vi "SetMeasBand.vi"(6 "Legacy (f)?":bool, 8 "error in (no error)":errorcluster, 10 "Band Index":u32) -> (0 "error out":errorcluster)   [LabVIEW 2011]
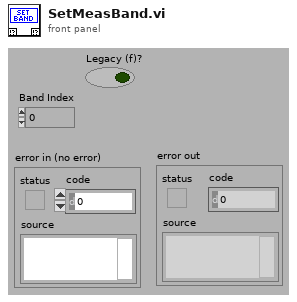
[diagram p1: front panel]
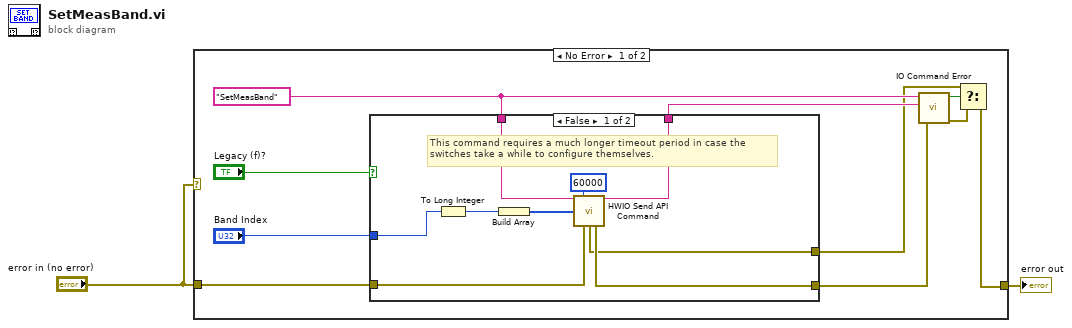
[diagram p0: block diagram]
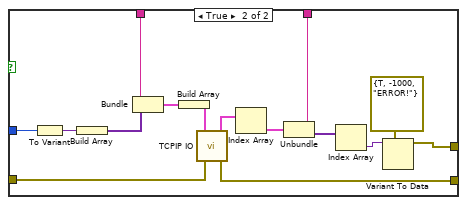
[diagram p2: hidden frame]
diagram:
  n1 = case shown="No Error" "error in (no error)" {
    tunnel: "error in (no error)" -> [w11 w37]
    tunnel: [w4 w37] -> w2
    frame No Error {
      w9 = "SetMeasBand"
      n2 = case shown="False" "Legacy (f)?" {
        tunnel: "Band Index" -> [w21 w36]
        tunnel: w11 -> [w20 w33]
        tunnel: [w19 w31] -> w10
        tunnel: w9 -> [w17 w30]
        tunnel: [w18 w26] -> w8
        tunnel: [w14 w23] -> w5
        frame False {
          # "This command requires a much longer timeout period in case the\nswitches take a while to configure themselves."
          n3 = To Long Integer(number=w21) -> (32bit integer=w15:i32)
          n4 = Build Array(w15) -> (w16:i32[])
          n5 = call "HWIO Send API Command.vi"("Action"=w17, "Timeout ms (5000)"=60000 ("Timeout ms (10000)"), "Integer"=w16, "error in (no error)"=w20) -> ("Action out"=w18:string, "HWError"=w14:errorcluster, "error out"=w19:errorcluster)  [unwired: 4 in, 5 out]
        }
        frame True {
          n6 = To Variant(anything=w36) -> (Variant=w35:variant)
          n7 = Build Array(w35) -> (w34:variant[])
          n8 = Bundle(w30, w34) -> (w32:cluster{string, variant[]})  [unwired: 1 out]
          n9 = Build Array(w32) -> (w29:cluster{string, variant[]}[])
          n10 = call "TCPIP IO.vi"("error in (no error)"=w33, "Commands"=w29) -> ("error out"=w31:errorcluster, "Responses"=w27:cluster{string, variant[]}[])  [unwired: 1 in, 3 out]
          n11 = Index Array(array=w27) -> (element=w28:cluster{string, variant[]})  [unwired: 1 in]
          n12 = Unbundle(w28) -> (w26:string, w24:variant[])
          n13 = Index Array(array=w24) -> (element=w25:variant)  [unwired: 1 in]
          n14 = Variant To Data(type=errorcluster {"status"=TRUE, "code"=-1000, "source"="ERROR!"} ("error out"), Variant=w25) -> (data=w23:errorcluster)  [unwired: 1 in, 1 out]
        }
      }
      n15 = call "IO Command Error.vi"("error in (no error)"=w10, "Command Returned (\"\")"=w8, "Command Sent (\"\")"=w9) -> ("error out"=w6:errorcluster, "HW ERR?"=w7:bool)  [unwired: 3 out]
      n16 = Select(t=w5, s=w7, f=w6) -> (s? t:f=w4:errorcluster)
    }
    frame Error {
    }
  }
  "error out" <- w2
